vi "Reset.vi"(8 "error in (no error)":errorcluster, 11 "ArrayController in":refnum<class "ArrayController.lvclass">) -> (0 "error out":errorcluster, 3 "ArrayController out":refnum<class "ArrayController.lvclass">)   [LabVIEW 2018, in "ArrayController.lvclass"]
uses:
  ArrayController.lvclass
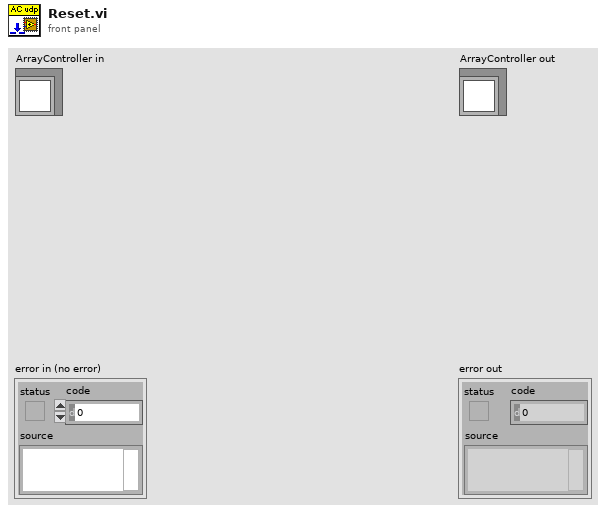
[diagram p1: front panel]
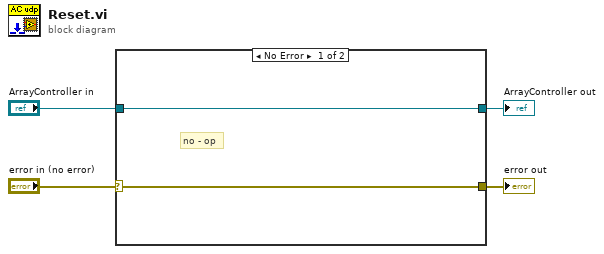
[diagram p0: block diagram]
diagram:
  n1 = case shown="No Error" "error in (no error)" {
    selector: "error in (no error)" -> [w5 w8]
    tunnel: [w5 w8] -> w3
    tunnel: [w6 w7] -> w1
    tunnel: "ArrayController in" -> [w6 w7]
    frame No Error {
      # "no - op"
    }
    frame Error {
    }
  }
  "error out" <- w3
  "ArrayController out" <- w1
